vi "EventStructureDO.vi"() -> ()   [LabVIEW 2020]
uses:
  <instrlib>/HandsOnPi2040/Public/DigOuts.ctl
  <instrlib>/HandsOnPi2040/HandsOnPi2040.lvlib
panel:
  in  "DO Value 4":bool
  in  "DO Value 3":bool
  in  "DO Value 2":bool
  in  "DO Value":bool
  in  "stop":bool
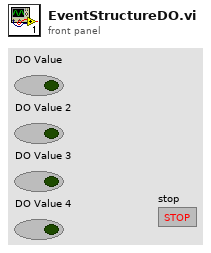
[diagram p1: front panel]
types:
  T1 = typedef "HandsOnPi2040.lvlib/DigOuts.ctl" = enum16{"No DO - Error", "DO1 (GPIO2)", "DO2 (GPIO3)", "DO3 (GPIO4)", "DO4 (GPIO5)", "BEEP (GPIO6)"}
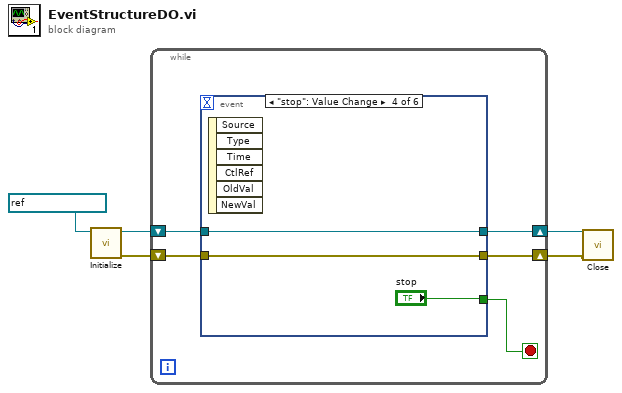
[diagram p0: block diagram]
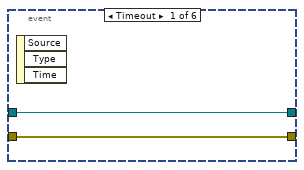
[diagram p2: hidden frame]
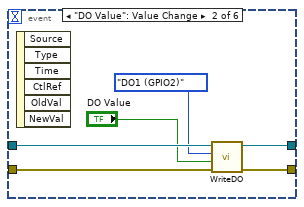
[diagram p3: hidden frame]
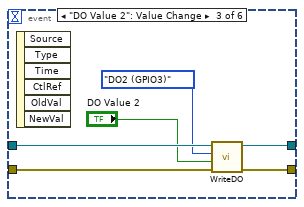
[diagram p4: hidden frame]
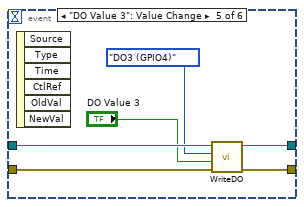
[diagram p5: hidden frame]
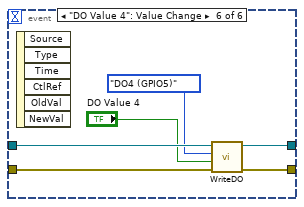
[diagram p6: hidden frame]
diagram:
  n1 = call <instrlib>:"Initialize.vi"("VISA resource name"=refnum<visa-resource-name> "ASRL1::INSTR") -> ("error out"=w3:errorcluster, "VISA resource name out"=w4:refnum<visa-resource-name>)  [unwired: 8 in, 1 out]
  n2 = while {
    shift-right: [w8] -> w2
    shift-left: w4 -> [w10]
    shift-right: [w7] -> w1
    shift-left: w3 -> [w9]
    stop <- w6 stop-if-true
    n3 = event shown="[3] \"stop\": Value Change" {
      selector: _ -> [_ _ _ _ _ _]
      dyn-events: _ -> [_ _ _ _ _ _]
      timeout: _ -> [_ _ _ _ _ _]
      tunnel: w10 -> [w12 w16 w22 w27 w31 w37]
      tunnel: w9 -> [w11 w14 w20 w26 w29 w35]
      tunnel: [w12 w18 w24 w27 w33 w39] -> w8
      tunnel: [w11 w17 w23 w26 w32 w38] -> w7
      tunnel: [_ _ _ "stop" _ _] -> w6
      event Timeout {
        n4 = event-data() -> ()  [unwired: 1 in, 3 out]
      }
      event "DO Value": Value Change {
        n5 = event-data() -> ()  [unwired: 1 in, 6 out]
        n6 = call <instrlib>:"WriteDO.vi"("error in (no error)"=w14, "DO Value (True)"="DO Value", "Output"=DigOuts."DO1 (GPIO2)", "VISA resource name"=w16) -> ("error out"=w17:errorcluster, "VISA resource name out"=w18:refnum<visa-resource-name>)  [unwired: 6 in]
      }
      event "DO Value 2": Value Change {
        n7 = event-data() -> ()  [unwired: 1 in, 6 out]
        n8 = call <instrlib>:"WriteDO.vi"("error in (no error)"=w20, "DO Value (True)"="DO Value 2", "Output"=DigOuts."DO2 (GPIO3)", "VISA resource name"=w22) -> ("error out"=w23:errorcluster, "VISA resource name out"=w24:refnum<visa-resource-name>)  [unwired: 6 in]
      }
      event "stop": Value Change {
        n9 = event-data() -> ()  [unwired: 1 in, 6 out]
      }
      event "DO Value 3": Value Change {
        n10 = event-data() -> ()  [unwired: 1 in, 6 out]
        n11 = call <instrlib>:"WriteDO.vi"("error in (no error)"=w29, "DO Value (True)"="DO Value 3", "Output"=DigOuts."DO3 (GPIO4)", "VISA resource name"=w31) -> ("error out"=w32:errorcluster, "VISA resource name out"=w33:refnum<visa-resource-name>)  [unwired: 6 in]
      }
      event "DO Value 4": Value Change {
        n12 = event-data() -> ()  [unwired: 1 in, 6 out]
        n13 = call <instrlib>:"WriteDO.vi"("error in (no error)"=w35, "DO Value (True)"="DO Value 4", "Output"=DigOuts."DO4 (GPIO5)", "VISA resource name"=w37) -> ("error out"=w38:errorcluster, "VISA resource name out"=w39:refnum<visa-resource-name>)  [unwired: 6 in]
      }
    }
  }
  n14 = call <instrlib>:"Close.vi"("error in (no error)"=w1, "VISA resource name"=w2) -> ()  [unwired: 9 in, 1 out]
